vi "Global_Config.vi"() -> ()   [LabVIEW 2011]
panel:
  in  "ESPELHO cluster":T1={"Mec ID"="1", "VISA Mec"="COM6", "Mec PosLimit"="131", "Mec NegLimit"="-1", "Mec Factor"=8000.0, "Mec Speed"=2.5, "Mec Acceleration"=133.0, "MecOffset"="0", "MecTargets"=[0.0, 4.0, 34.0, 64.5, 95.0, 125.5], "MecEnabled"=TRUE, "Mec Target"=0.0, "FLAG"=FALSE}
  in  "FENDA cluster":T1={"Mec ID"="1", "VISA Mec"="COM6", "Mec PosLimit"="131", "Mec NegLimit"="-1", "Mec Factor"=8000.0, "Mec Speed"=2.5, "Mec Acceleration"=133.0, "MecOffset"="0", "MecTargets"=[0.0, 4.0, 34.0, 64.5, 95.0, 125.5], "MecEnabled"=TRUE, "Mec Target"=0.0, "FLAG"=FALSE}
  in  "PRISMA cluster":T1={"Mec ID"="1", "VISA Mec"="COM6", "Mec PosLimit"="131", "Mec NegLimit"="-1", "Mec Factor"=8000.0, "Mec Speed"=2.5, "Mec Acceleration"=133.0, "MecOffset"="0", "MecTargets"=[0.0, 4.0, 34.0, 64.5, 95.0, 125.5], "MecEnabled"=TRUE, "Mec Target"=0.0, "FLAG"=FALSE}
  out "SHUTTERDATA2":cluster{"LastPosition":string, "Target":string}
  out "FOCUSDATA2":cluster{"LastPosition":string, "Target":string}
  out "MASKDATA2":cluster{"LastPosition":string, "Target":string}
  out "LENSDATA2":cluster{"LastPosition":string, "Target":string}
  out "FILTERDATA2":cluster{"LastPosition":string, "Target":string}
  out "SPECMODEDATA":T2
  out "GRATINGDATA":T2
  out "SHUTTERDATA":T2
  out "FOCUSDATA":T2
  out "MASKDATA":T2
  out "SPECMODEDATA2":T3
  out "GRATINGDATA2":T4
  out "LENSDATA":T2
  out "FILTERDATA":T2
  in  "FLAGS ACTIVE":bool[](array[boolean])=[TRUE, TRUE, TRUE, TRUE, TRUE, TRUE, TRUE, TRUE]
  in  "CAMERA cluster":T1={"Mec ID"="1", "VISA Mec"="COM6", "Mec PosLimit"="131", "Mec NegLimit"="-1", "Mec Factor"=8000.0, "Mec Speed"=2.5, "Mec Acceleration"=133.0, "MecOffset"="0", "MecTargets"=[0.0, 4.0, 34.0, 64.5, 95.0, 125.5], "MecEnabled"=TRUE, "Mec Target"=0.0, "FLAG"=FALSE}
  in  "GRATING cluster":T1={"Mec ID"="1", "VISA Mec"="COM6", "Mec PosLimit"="131", "Mec NegLimit"="-1", "Mec Factor"=8000.0, "Mec Speed"=2.5, "Mec Acceleration"=133.0, "MecOffset"="0", "MecTargets"=[0.0, 4.0, 34.0, 64.5, 95.0, 125.5], "MecEnabled"=TRUE, "Mec Target"=0.0, "FLAG"=FALSE}
  in  "FOCUS cluster":T1={"Mec ID"="1", "VISA Mec"="COM6", "Mec PosLimit"="131", "Mec NegLimit"="-1", "Mec Factor"=8000.0, "Mec Speed"=2.5, "Mec Acceleration"=133.0, "MecOffset"="0", "MecTargets"=[0.0, 4.0, 34.0, 64.5, 95.0, 125.5], "MecEnabled"=TRUE, "Mec Target"=0.0, "FLAG"=FALSE}
  in  "SHUTTER cluster":T1={"Mec ID"="1", "VISA Mec"="COM6", "Mec PosLimit"="131", "Mec NegLimit"="-1", "Mec Factor"=8000.0, "Mec Speed"=2.5, "Mec Acceleration"=133.0, "MecOffset"="0", "MecTargets"=[0.0, 4.0, 34.0, 64.5, 95.0, 125.5], "MecEnabled"=TRUE, "Mec Target"=0.0, "FLAG"=FALSE}
  in  "RACK cluster":T1={"Mec ID"="1", "VISA Mec"="COM6", "Mec PosLimit"="131", "Mec NegLimit"="-1", "Mec Factor"=8000.0, "Mec Speed"=2.5, "Mec Acceleration"=133.0, "MecOffset"="0", "MecTargets"=[0.0, 4.0, 34.0, 64.5, 95.0, 125.5], "MecEnabled"=TRUE, "Mec Target"=0.0, "FLAG"=FALSE}
  in  "PUSHPULL cluster":T1={"Mec ID"="1", "VISA Mec"="COM6", "Mec PosLimit"="131", "Mec NegLimit"="-1", "Mec Factor"=8000.0, "Mec Speed"=2.5, "Mec Acceleration"=133.0, "MecOffset"="0", "MecTargets"=[0.0, 4.0, 34.0, 64.5, 95.0, 125.5], "MecEnabled"=TRUE, "Mec Target"=0.0, "FLAG"=FALSE}
  in  "MASK cluster":T1={"Mec ID"="1", "VISA Mec"="COM6", "Mec PosLimit"="131", "Mec NegLimit"="-1", "Mec Factor"=8000.0, "Mec Speed"=2.5, "Mec Acceleration"=133.0, "MecOffset"="0", "MecTargets"=[0.0, 4.0, 34.0, 64.5, 95.0, 125.5], "MecEnabled"=TRUE, "Mec Target"=0.0, "FLAG"=FALSE}
  in  "LENS cluster":T1={"Mec ID"="1", "VISA Mec"="COM6", "Mec PosLimit"="131", "Mec NegLimit"="-1", "Mec Factor"=8000.0, "Mec Speed"=2.5, "Mec Acceleration"=133.0, "MecOffset"="0", "MecTargets"=[0.0, 4.0, 34.0, 64.5, 95.0, 125.5], "MecEnabled"=TRUE, "Mec Target"=0.0, "FLAG"=FALSE}
  in  "FILTER cluster":T1={"Mec ID"="1", "VISA Mec"="COM6", "Mec PosLimit"="131", "Mec NegLimit"="-1", "Mec Factor"=8000.0, "Mec Speed"=2.5, "Mec Acceleration"=133.0, "MecOffset"="0", "MecTargets"=[0.0, 4.0, 34.0, 64.5, 95.0, 125.5], "MecEnabled"=TRUE, "Mec Target"=0.0, "FLAG"=FALSE}
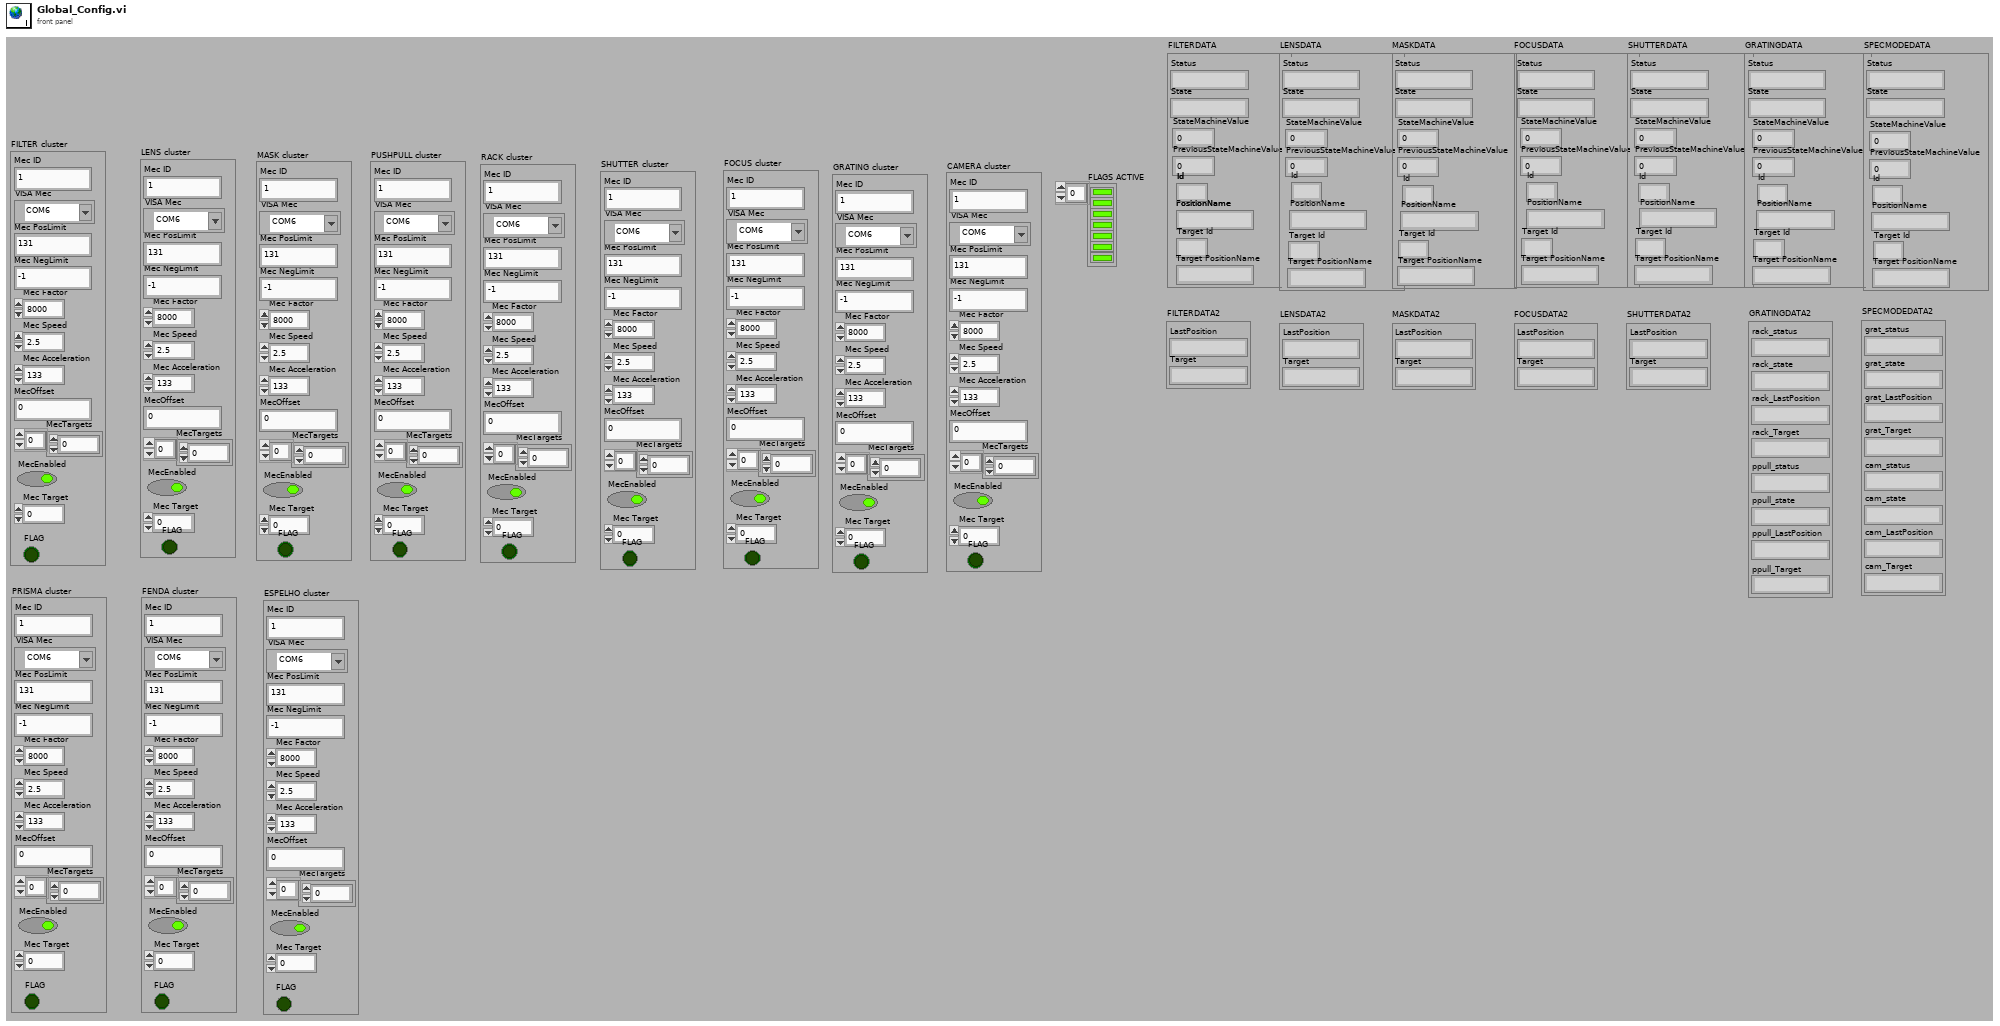
[diagram p1: front panel]
types:
  T1 = cluster{"Mec ID":string, "VISA Mec":refnum<visa-resource-name>, "Mec PosLimit":string, "Mec NegLimit":string, "Mec Factor":dbl, "Mec Speed":dbl, "Mec Acceleration":dbl, "MecOffset":string, "MecTargets":dbl[], "MecEnabled":bool, "Mec Target":dbl, "FLAG":bool}
  T2 = cluster{"Status":string, "State":string, "StateMachineValue":i32, "PreviousStateMachineValue":i32, "Id":string, "PositionName":string, "Target Id":string, "Target PositionName":string}
  T3 = cluster{"grat_status":string, "grat_state":string, "grat_LastPosition":string, "grat_Target":string, "cam_status":string, "cam_state":string, "cam_LastPosition":string, "cam_Target":string}
  T4 = cluster{"rack_status":string, "rack_state":string, "rack_LastPosition":string, "rack_Target":string, "ppull_status":string, "ppull_state":string, "ppull_LastPosition":string, "ppull_Target":string}
diagram:
